vi "LoadTSConfigFile.vi"(0 "Sequence path":path=path "C:/Func Jobs/SnapOn/modisEdge/Scanner/Test Sequence/ModisEdgeScanner.ini", 5 "file name":string="modisEdgeScanner.ini", 11 "error in (no error)":errorcluster) -> (1 "appended path":path, 2 "PS1_COMPort":i32, 3 "InterlockDevice":string, 4 "SnapOnTestScriptFile":string, 6 "UUT_COMPort":i32, 8 "DMM_COMPort":i32, 10 "ResultsFolder":string, 12 "FixtureID":string, 13 "PS2_COMPort":i32, 14 "DAQDevice":string, 15 "error out":errorcluster={"status"=TRUE, "code"=7, "source"="NI_LVConfig.lvlib:Load.vi"})   [LabVIEW 2015]
doc: "Use this template to build a VI to use as a subVI."
uses:
  <vilib>/Utility/config.llb/Read Key (String).vi
  <vilib>/Utility/config.llb/NI_LVConfig.lvlib
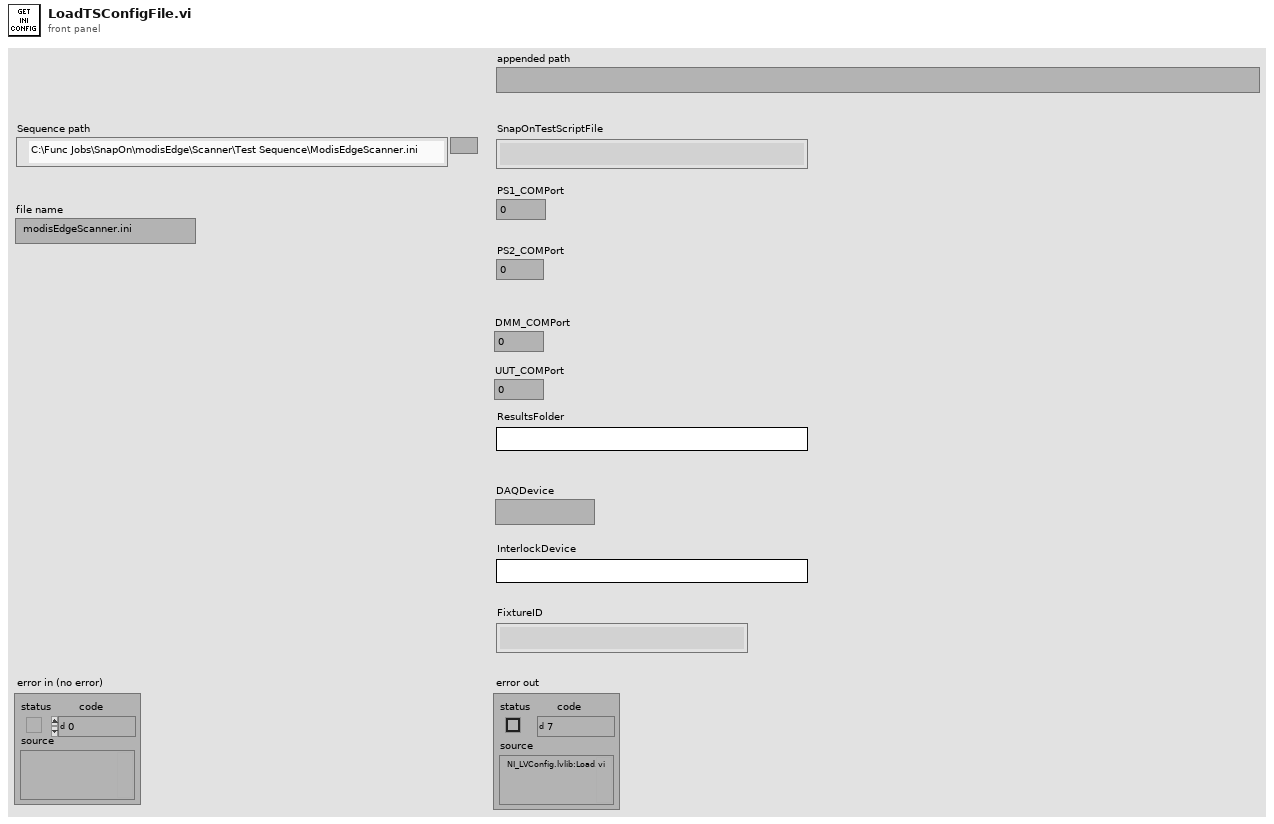
[diagram p1: front panel]
types:
  T1 = typedef "NI_LVConfig.lvlib/Config Data RefNum.ctl" = refnum<k1>
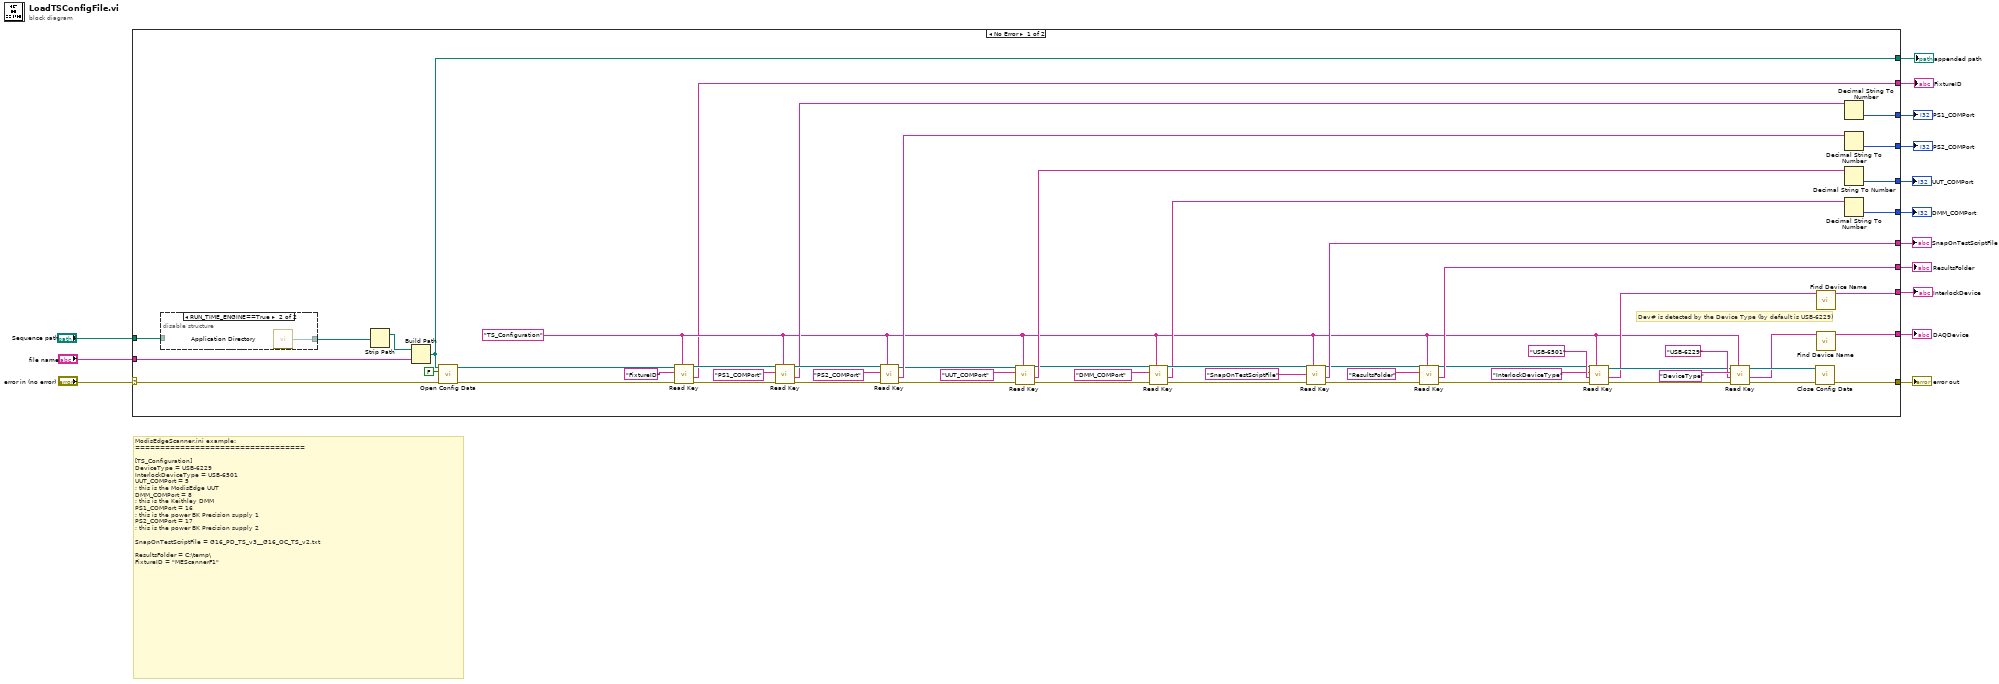
[diagram p0: block diagram]
diagram:
  # "ModisEdgeScanner.ini example:\n==================================\n\n[TS_Configuration]\nDeviceType = USB-6229\nInterlockDeviceType = USB-6501\nUUT_COMPort = 5 \t\n; this is the ModisEdge UUT\nDMM_COMPort = 8\t\t\n; this is the Keithley DMM\nPS1_COMPort = 16\t\n; this is the power BK Precision supply 1 \nPS2_COMPort = 17\n; this is the power BK Precision supply 2\n\nSnapOnTestScriptFile = G16_PD_TS_v3__G16_OC_TS_v2.txt\n\nResultsFolder = C:\\temp\\\nFixtureID = \"MEScannerF1\""
  n1 = case shown="No Error" "error in (no error)" {
    selector: "error in (no error)" -> [w66 w72]
    tunnel: [w63 w72] -> w13
    tunnel: [w67 _] -> w12
    tunnel: [w64 _] -> w11
    tunnel: [w59 _] -> w10
    tunnel: "Sequence path" -> [w22 _]
    tunnel: [w53 _] -> w9
    tunnel: [w45 _] -> w8
    tunnel: [w38 _] -> w7
    tunnel: "file name" -> [w36 _]
    tunnel: [w30 _] -> w5
    tunnel: [w29 _] -> w4
    tunnel: [w24 _] -> w3
    tunnel: [w15 _] -> w1
    frame No Error {
      w17 = "TS_Configuration" ("key")
      # "Dev# is detected by the Device Type (by default is USB-6229)"
      n2 = disable-structure shown="RUN_TIME_ENGINE==True" {
        disable-tunnel: [w70 w71] -> w23
        disable-tunnel: w22 -> [w70 _]
        frame condition #0 (active) {
        }
        frame condition #1 {
          n3 = call <vilib>:"Application Directory.vi"() -> ("Application Directory"=w71:path)
        }
      }
      n4 = Strip Path(path=w23) -> (stripped path=w37:path)  [unwired: 1 out]
      n5 = Build Path(base path=w37, name or relative path=w36) -> (appended path=w24:path)
      n6 = call <vilib>:"Open Config Data.vi"("error in (no error)"=w66, "create file if necessary (T)"=FALSE, "configuration file path"=w24) -> ("error out"=w18:errorcluster, "refnum"=w20:T1)  [unwired: 6 in, 1 out]
      n7 = call-poly <vilib>:"Read Key.vi"("section"=w17, "error in (no error)"=w18, "key"="FixtureID", "refnum"=w20) -> ("error out"=w21:errorcluster, "value"=w15:string, "refnum out"=w19:T1)  [unwired: 4 in, 1 out]
      n8 = call-poly <vilib>:"Read Key.vi"("section"=w17, "error in (no error)"=w21, "key"="PS1_COMPort", "refnum"=w19) -> ("error out"=w34:errorcluster, "value"=w27:string, "refnum out"=w33:T1)  [unwired: 4 in, 1 out]
      n9 = call-poly <vilib>:"Read Key.vi"("section"=w17, "error in (no error)"=w34, "key"="PS2_COMPort", "refnum"=w33) -> ("error out"=w28:errorcluster, "value"=w26:string, "refnum out"=w25:T1)  [unwired: 4 in, 1 out]
      n10 = call-poly <vilib>:"Read Key.vi"("section"=w17, "error in (no error)"=w28, "key"="UUT_COMPort", "refnum"=w25) -> ("error out"=w41:errorcluster, "value"=w65:string, "refnum out"=w43:T1)  [unwired: 4 in, 1 out]
      n11 = call-poly <vilib>:"Read Key.vi"("section"=w17, "error in (no error)"=w41, "key"="DMM_COMPort", "refnum"=w43) -> ("error out"=w40:errorcluster, "value"=w39:string, "refnum out"=w42:T1)  [unwired: 4 in, 1 out]
      n12 = call-poly <vilib>:"Read Key.vi"("section"=w17, "error in (no error)"=w40, "key"="SnapOnTestScriptFile", "refnum"=w42) -> ("error out"=w60:errorcluster, "value"=w67:string, "refnum out"=w61:T1)  [unwired: 4 in, 1 out]
      n13 = call-poly <vilib>:"Read Key.vi"("section"=w17, "error in (no error)"=w60, "key"="ResultsFolder", "refnum"=w61) -> ("error out"=w50:errorcluster, "value"=w59:string, "refnum out"=w48:T1)  [unwired: 4 in, 1 out]
      n14 = call-poly <vilib>:"Read Key.vi"("section"=w17, "error in (no error)"=w50, "default value"="USB-6501", "key"="InterlockDeviceType", "refnum"=w48) -> ("error out"=w49:errorcluster, "value"=w46:string, "refnum out"=w47:T1)  [unwired: 3 in, 1 out]
      n15 = call-poly <vilib>:"Read Key.vi"("section"=w17, "error in (no error)"=w49, "default value"="USB-6229", "key"="DeviceType", "refnum"=w47) -> ("error out"=w57:errorcluster, "value"=w54:string, "refnum out"=w56:T1)  [unwired: 3 in, 1 out]
      n16 = call <vilib>:"Close Config Data.vi"("error in (no error)"=w57, "refnum"=w56) -> ("error out"=w63:errorcluster)  [unwired: 8 in, 1 out]
      n17 = call "Find Device Name.vi"("Device Type"=w46) -> ("Device Name"=w45:string)  [unwired: 10 in]
      n18 = call "Find Device Name.vi"("Device Type"=w54) -> ("Device Name"=w53:string)  [unwired: 10 in]
      n19 = Decimal String To Number(string=w27) -> (number=w30:i32)  [unwired: 2 in, 1 out]
      n20 = Decimal String To Number(string=w26) -> (number=w29:i32)  [unwired: 2 in, 1 out]
      n21 = Decimal String To Number(string=w65) -> (number=w64:i32)  [unwired: 2 in, 1 out]
      n22 = Decimal String To Number(string=w39) -> (number=w38:i32)  [unwired: 2 in, 1 out]
    }
    frame Error {
    }
  }
  "error out" <- w13
  "SnapOnTestScriptFile" <- w12
  "UUT_COMPort" <- w11
  "ResultsFolder" <- w10
  "DAQDevice" <- w9
  "InterlockDevice" <- w8
  "DMM_COMPort" <- w7
  "PS1_COMPort" <- w5
  "PS2_COMPort" <- w4
  "appended path" <- w3
  "FixtureID" <- w1
